vi "Read State.vi"(8 "error in (no error)":errorcluster, 11 "Container State in":refnum<class "Container State.lvclass">) -> (0 "error out":errorcluster, 2 "State.lvlib:State.lvclass":refnum<class "State.lvclass">, 3 "Container State out":refnum<class "Container State.lvclass">)   [LabVIEW 2024]
uses:
  Container State.lvclass
  State/State.lvclass
  Container State.lvclass/Container State.ctl
  C:/Users/uspoaotto/OneDrive - Oregon Tool/Desktop/working copies/stateMachineActor/src/State Machine/State/State/State.lvclass
  C:/Users/uspoaotto/OneDrive - Oregon Tool/Desktop/working copies/stateMachineActor/src/State Machine/State/Container State/Container State.lvclass
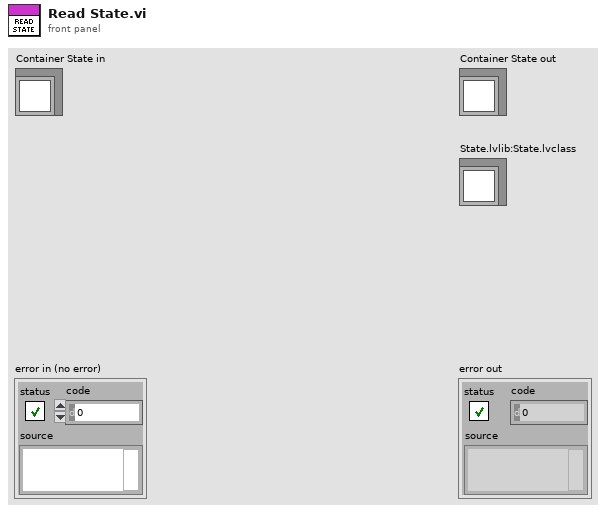
[diagram p1: front panel]
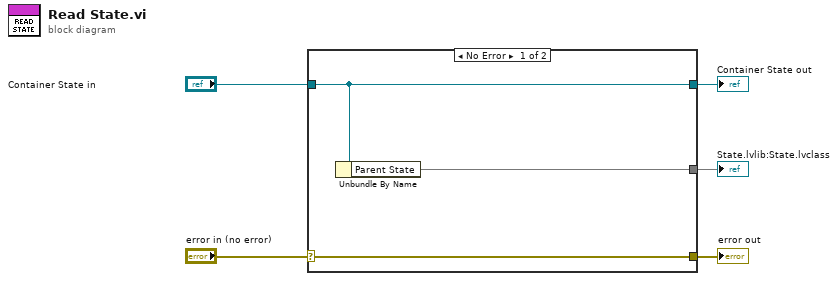
[diagram p0: block diagram]
diagram:
  n1 = case shown="No Error" "error in (no error)" {
    selector: "error in (no error)" -> [w8 w9]
    tunnel: [w8 w9] -> w4
    tunnel: [w7 w10] -> w2
    tunnel: "Container State in" -> [w7 w10]
    tunnel: [w6 _] -> w1
    frame No Error {
      n2 = Unbundle By Name(w7) -> ("Parent State"=w6)
    }
    frame Error {
    }
  }
  "error out" <- w4
  "Container State out" <- w2
  "State.lvlib:State.lvclass" <- w1
